vi "MenuSelection(User).vi"(6 "User events":T8, 7 "Clipboard":refnum<vi>, 8 "error in":errorcluster {"code" min=0 max=0}, 10 "ItemTag":string, 11 "Data in":T1={"Class"={"Ants"=refnum, "Layer"=refnum, "Templates"=refnum, "Icon"=refnum, "Glyph"=refnum, "Settings"=refnum, "Tools"=refnum}, "Ref"={"Add Layer"=refnum, "Remove Layer"=refnum, "Line Text"=[], "Body Text Spec"=refnum, "DNL_Font"=refnum, "glyph path str"=refnum, "templates path str"=refnum, "Arrow Up"=refnum, "Arrow Down"=refnum, "IE VI Ref"=refnum, "Glyphs tree"=refnum, "Templates tree"=refnum, "Layer Icon Text"=refnum, "Layer Template"=refnum, "Body Text"=refnum, "Search Templates"=refnum, "TextMarker"=refnum, "Tab Control"=refnum, "Search Glyphs"=refnum, "Line Color"=refnum, "DNL_Glyphs []"=refnum, "Fill Color"=refnum, "Tools"=refnum, "Icon"=refnum, "Preview"=refnum, "Ants"=refnum, "Terminals"=refnum, "menu reference"=refnum, "LayerNames"=[], "GlyphLoadAnimation"=refnum, "TemplateLoadAnimation"=refnum, "refreshGlyphs"=refnum, "refreshTemplates"=refnum}, "Support"={"AntsRect"={"left"=0, "top"=0, "right"=0, "bottom"=0}, "Mouse Move Coords"={"Horizontal"=0, "Vertical"=0}, "Mouse Down Coords"={"Horizontal"=0, "Vertical"=0}, "Temp Coord"={"Horizontal"=0, "Vertical"=0}, "Action"=enum."Default", "Edge Color"=4914962, "Fill Color"=16860, "Mouse Down?"=FALSE, "Draft Mode?"=FALSE, "Temp Icon"=bytes[3102], "CTRL Pressed"=FALSE, "Move Selection?"=FALSE, "AntsRect Orig"={"left"=0, "top"=0, "right"=0, "bottom"=0}, "Text"="", "TM Set?"=FALSE, "Mouse inside icon?"=FALSE, "Tool (old value)"=0, "Pencil Move Color"=0, "Swap Colors?"=FALSE, "Shift pressed?"=FALSE}}) -> (0 "error out":errorcluster {"code" min=0 max=0}, 3 "Data out":T1={"Class"={"Ants"=refnum, "Layer"=refnum, "Templates"=refnum, "Icon"=refnum, "Glyph"=refnum, "Settings"=refnum, "Tools"=refnum}, "Ref"={"Add Layer"=refnum, "Remove Layer"=refnum, "Line Text"=[], "Body Text Spec"=refnum, "DNL_Font"=refnum, "glyph path str"=refnum, "templates path str"=refnum, "Arrow Up"=refnum, "Arrow Down"=refnum, "IE VI Ref"=refnum, "Glyphs tree"=refnum, "Templates tree"=refnum, "Layer Icon Text"=refnum, "Layer Template"=refnum, "Body Text"=refnum, "Search Templates"=refnum, "TextMarker"=refnum, "Tab Control"=refnum, "Search Glyphs"=refnum, "Line Color"=refnum, "DNL_Glyphs []"=refnum, "Fill Color"=refnum, "Tools"=refnum, "Icon"=refnum, "Preview"=refnum, "Ants"=refnum, "Terminals"=refnum, "menu reference"=refnum, "LayerNames"=[], "GlyphLoadAnimation"=refnum, "TemplateLoadAnimation"=refnum, "refreshGlyphs"=refnum, "refreshTemplates"=refnum}, "Support"={"AntsRect"={"left"=0, "top"=0, "right"=0, "bottom"=0}, "Mouse Move Coords"={"Horizontal"=0, "Vertical"=0}, "Mouse Down Coords"={"Horizontal"=0, "Vertical"=0}, "Temp Coord"={"Horizontal"=0, "Vertical"=0}, "Action"=enum."Default", "Edge Color"=4914962, "Fill Color"=16860, "Mouse Down?"=FALSE, "Draft Mode?"=FALSE, "Temp Icon"=bytes[3102], "CTRL Pressed"=FALSE, "Move Selection?"=FALSE, "AntsRect Orig"={"left"=0, "top"=0, "right"=0, "bottom"=0}, "Text"="", "TM Set?"=FALSE, "Mouse inside icon?"=FALSE, "Tool (old value)"=0, "Pencil Move Color"=0, "Swap Colors?"=FALSE, "Shift pressed?"=FALSE}})   [LabVIEW 2021]
uses:
  <resource>/plugins/NIIconEditor/Controls/Global Data.ctl
  <resource>/plugins/NIIconEditor/Class/Ants/Ants.lvclass
  <resource>/plugins/NIIconEditor/Class/FakedArray/FakedArray.lvclass
  <vilib>/LabVIEW Icon API/lv_icon/Classes/Icon/Icon.lvclass
  <resource>/plugins/NIIconEditor/Class/Icon Library/Glyph.lvclass
  <resource>/plugins/NIIconEditor/Class/Settings/Settings.lvclass
  <resource>/plugins/NIIconEditor/Class/Tools/Tools Paint.lvclass
  <resource>/plugins/NIIconEditor/Controls/IE Classes.ctl
  <resource>/plugins/NIIconEditor/Controls/References Cluster.ctl
  <resource>/plugins/NIIconEditor/Controls/SupportClass.ctl
  <vilib>/Utility/miscctls.llb/LVPoint32TypeDef.ctl
  <resource>/plugins/NIIconEditor/Controls/SupportClass_Action.ctl
  <vilib>/LabVIEW Icon API/lv_icon/Controls/IEColor.ctl
  <vilib>/LabVIEW Icon API/lv_icon/Controls/Pathes.ctl
  <vilib>/LabVIEW Icon API/lv_icon/Controls/Graphic.ctl
  <vilib>/LabVIEW Icon API/lv_icon/Classes/Icon Framework/Icon Framework.lvclass
  <vilib>/LabVIEW Icon API/lv_icon/Classes/Layer/Layer.lvclass
  <vilib>/LabVIEW Icon API/lv_icon/Controls/Layer.ctl
  <resource>/plugins/NIIconEditor/Controls/Undo Redo Action.ctl
  <resource>/plugins/NIIconEditor/Controls/Tools.ctl
  <vilib>/LabVIEW Icon API/lv_icon/lv_icon.lvlib
panel:
  in  "Layer name":string="Clipboard"
  in  "glyph":string="Glyph name"
  in  "template":string="Template name"
  in  "Prompt":string="Save Glyph"
  in  "prompt":string="Save Icon Template"
  in  "LayerName":string="Merged Layers"
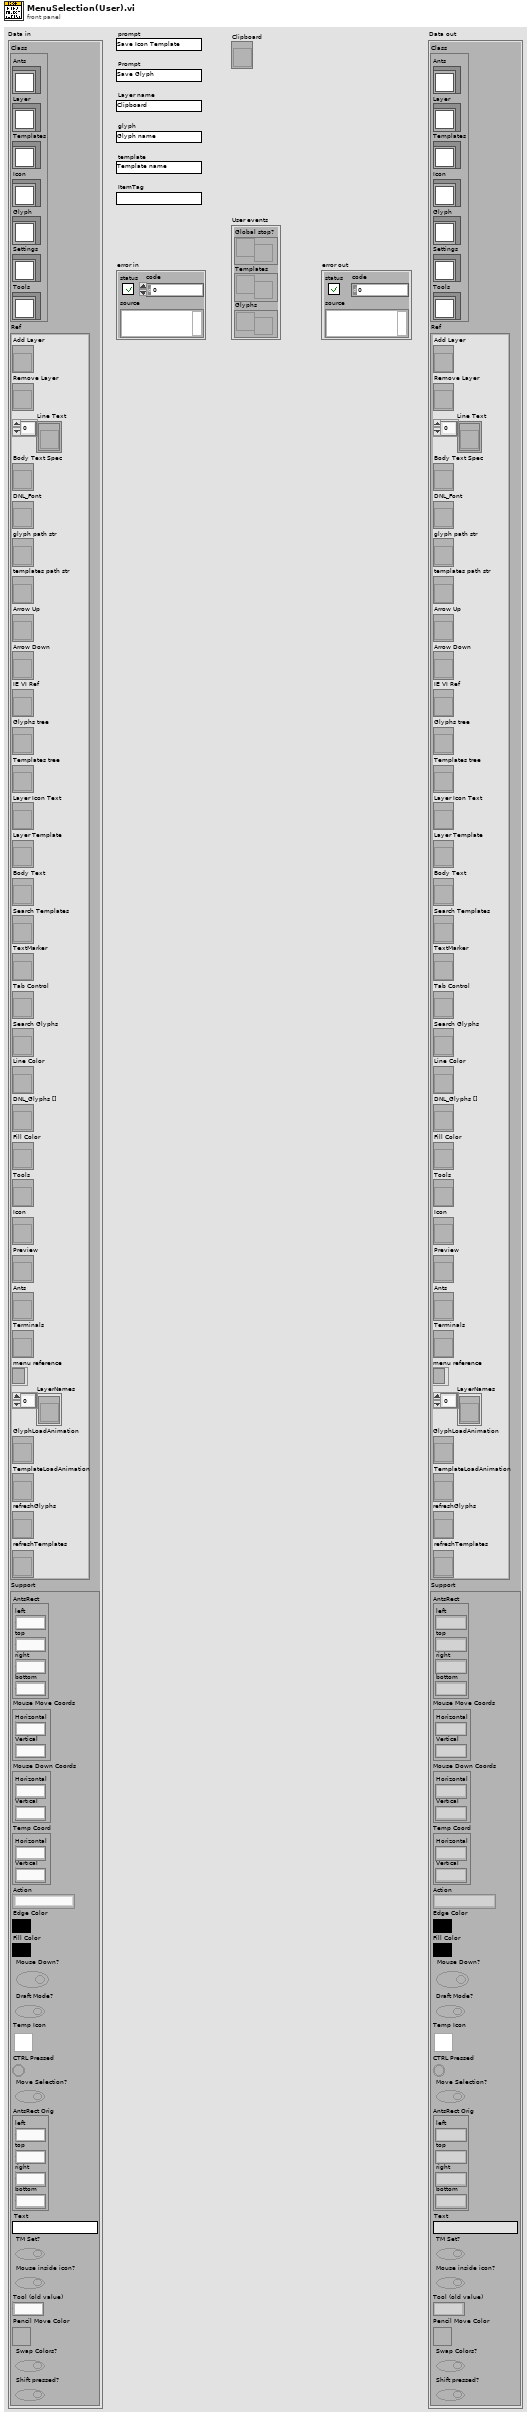
[diagram p1: front panel]
types:
  T1 = typedef "lv_icon.lvlib/Global Data.ctl" = cluster{"Class":T2, "Ref":T3, "Support":T4}
  T2 = typedef "IE Classes.ctl" = cluster{"Ants":refnum<class "Ants.lvclass">, "Layer":refnum<class "FakedArray.lvclass">, "Templates":refnum<class "FakedArray.lvclass">, "Icon":refnum<class "Icon.lvclass">, "Glyph":refnum<class "Glyph.lvclass">, "Settings":refnum<class "Settings.lvclass">, "Tools":refnum<class "Tools Paint.lvclass">}
  T3 = typedef "lv_icon.lvlib/References Cluster.ctl" = cluster{"Add Layer":refnum<vi>, "Remove Layer":refnum<vi>, "Line Text":refnum<vi>[], "Body Text Spec":refnum<vi>, "DNL_Font":refnum<vi>, "glyph path str":refnum<vi>, "templates path str":refnum<vi>, "Arrow Up":refnum<vi>, "Arrow Down":refnum<vi>, "IE VI Ref":refnum<vi>, "Glyphs tree":refnum<vi>, "Templates tree":refnum<vi>, "Layer Icon Text":refnum<vi>, "Layer Template":refnum<vi>, "Body Text":refnum<vi>, "Search Templates":refnum<vi>, "TextMarker":refnum<vi>, "Tab Control":refnum<vi>, "Search Glyphs":refnum<vi>, "Line Color":refnum<vi>, "DNL_Glyphs []":refnum<vi>, "Fill Color":refnum<vi>, "Tools":refnum<vi>, "Icon":refnum<vi>, "Preview":refnum<vi>, "Ants":refnum<vi>, "Terminals":refnum<vi>, "menu reference":refnum<k9>, "LayerNames":refnum<vi>[], "GlyphLoadAnimation":refnum<vi>, "TemplateLoadAnimation":refnum<vi>, "refreshGlyphs":refnum<vi>, "refreshTemplates":refnum<vi>}
  T4 = typedef "SupportClass.ctl" = cluster{"AntsRect":cluster{"left":i16, "top":i16, "right":i16, "bottom":i16}, "Mouse Move Coords":T5, "Mouse Down Coords":T5, "Temp Coord":T5, "Action":T6, "Edge Color":T7, "Fill Color":T7, "Mouse Down?":bool, "Draft Mode?":bool, "Temp Icon":picture, "CTRL Pressed":bool, "Move Selection?":bool, "AntsRect Orig":cluster{"left":i16, "top":i16, "right":i16, "bottom":i16}, "Text":string, "TM Set?":bool, "Mouse inside icon?":bool, "Tool (old value)":u32, "Pencil Move Color":u32, "Swap Colors?":bool, "Shift pressed?":bool}
  T5 = typedef "LVPoint32TypeDef.ctl" = cluster{"Horizontal":i32, "Vertical":i32}
  T6 = typedef "SupportClass_Action.ctl" = enum16{"Default", "Move Selection", "Glyph Library", "Tool"}
  T7 = typedef "IEColor.ctl" = u32
  T8 = cluster{"Global stop?":refnum<user-event>, "Templates":refnum<user-event>, "Glyphs":refnum<user-event>}
  T9 = typedef "Pathes.ctl" = enum16{"Root Path", "Icon Templates", "Icon Templates VI", "Icon Templates Lib", "Glyphs"}
  T10 = typedef "Graphic.ctl" = cluster{"Rectangle":cluster{"left":i16, "top":i16, "right":i16, "bottom":i16}, "Path":path, "Image":picture, "Filter":string, "FileName":string}
  T11 = typedef "Layer.ctl" = cluster{"LayerIcon":picture, "LayerName":string, "Opacity":u8, "Visibility?":bool}
  T12 = typedef "Undo Redo Action.ctl" = enum16{"Init", "Add", "Undo", "Redo", "Current State"}
  T13 = enum32{"Pencil", "Line", "Dropper", "Fill", "Rectangle", "Filled Rectangle", "Ellipse", "Filled Ellipse", "Eraser", "Text", "Select", "Move"}
  T14 = typedef "Tools.ctl" = enum32{"Pencil", "Line", "Dropper", "Fill", "Rectangle", "Filled Rectangle", "Ellipse", "Filled Ellipse", "Eraser", "Text", "Select", "Move"}
  T15 = typedef "imagedata.ctl" = cluster{"image type":i32, "image depth":i32, "image":u8[], "mask":u8[], "colors":u32[], "Rectangle":cluster{"left":i16, "top":i16, "right":i16, "bottom":i16}}
  T16 = typedef "Font.ctl" = string
  T17 = typedef "Alignment.ctl" = u16
  T18 = typedef "Font Size.ctl" = u8
  T19 = cluster{"Line 1 text":string, "Line 2 text":string, "Line 3 text":string, "Line 4 text":string, "Line 1 color":u32, "Line 2 color":u32, "Line 3 color":u32, "Line 4 color":u32, "Body Text Spec":cluster{"DNL_Font":T16, "Alignment":T17, "Size":T18}, "Center text vertically":bool, "Capitalize Text":bool}
  T20 = cluster{"left":i16, "top":i16, "right":i16, "bottom":i16}
  T21 = cluster{"Horizontal":i32, "Vertical":i32, "Vertical 2":i32, "Vertical 3":i32}
  T22 = cluster{"Left":i32, "Top":i32, "Right":i32, "Bottom":i32}
  T23 = typedef "Icon Editor Invoker Type.ctl" = enum32{"Unknown Icon Source", "VI Icon", "Library Icon (any library type)", "Palette icon", "Icon from App Method"}
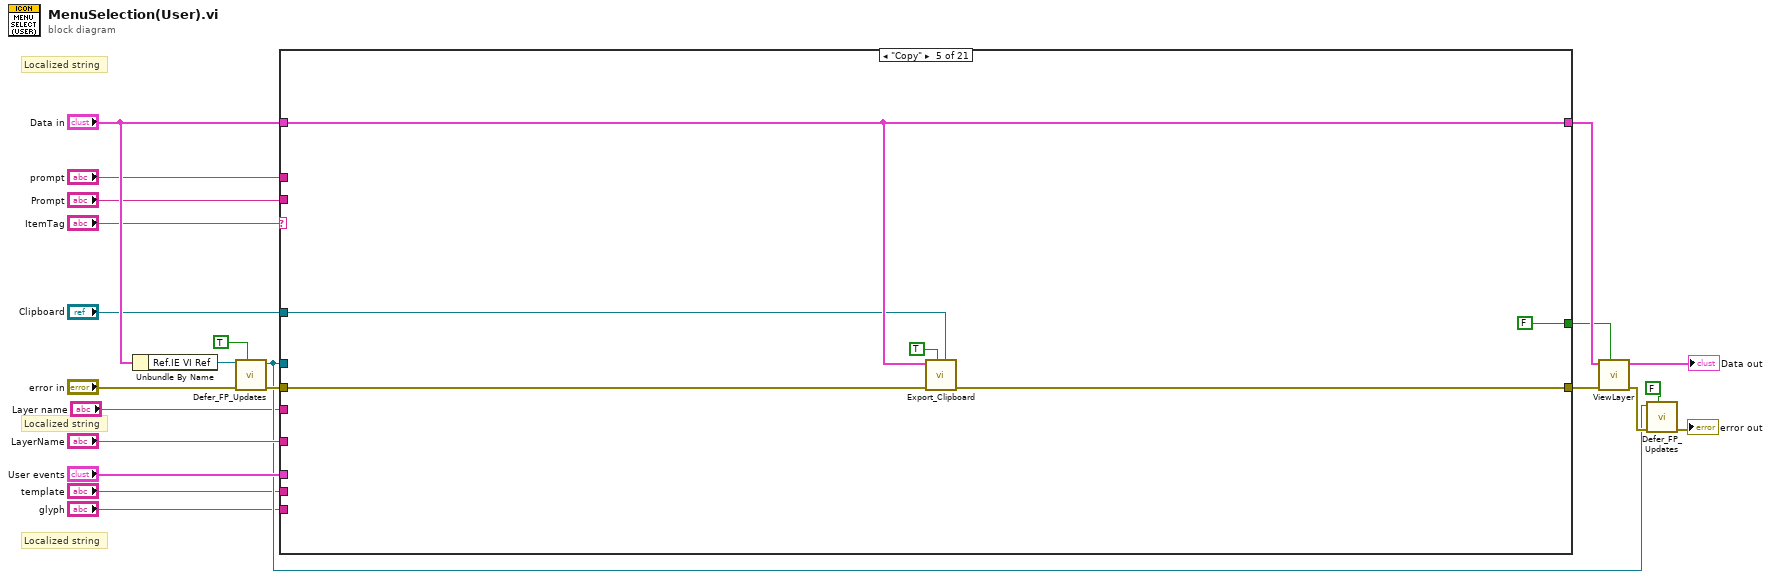
[diagram p0: block diagram]
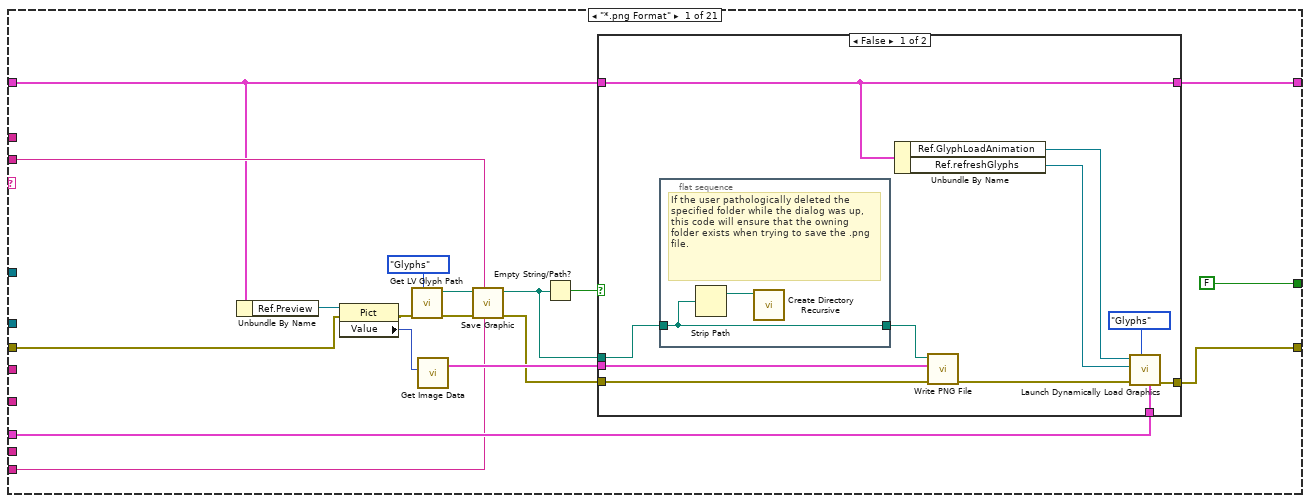
[diagram p2: hidden frame]
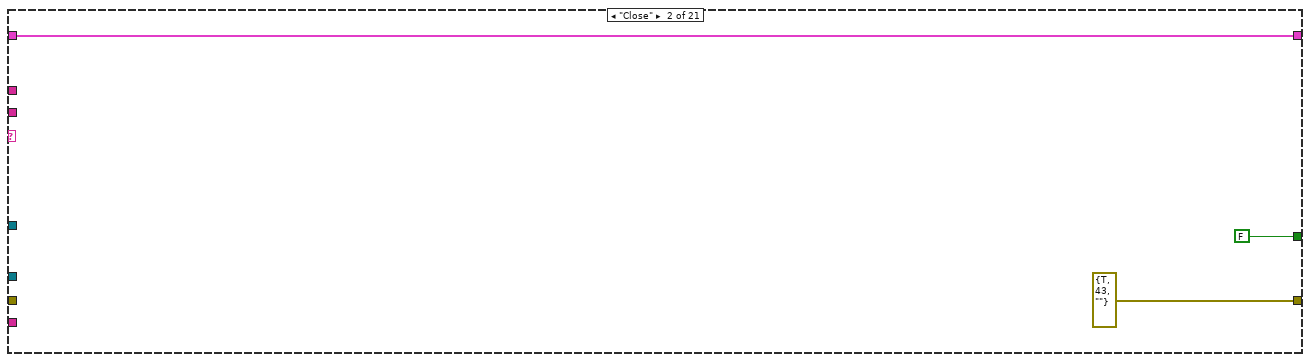
[diagram p4: hidden frame]
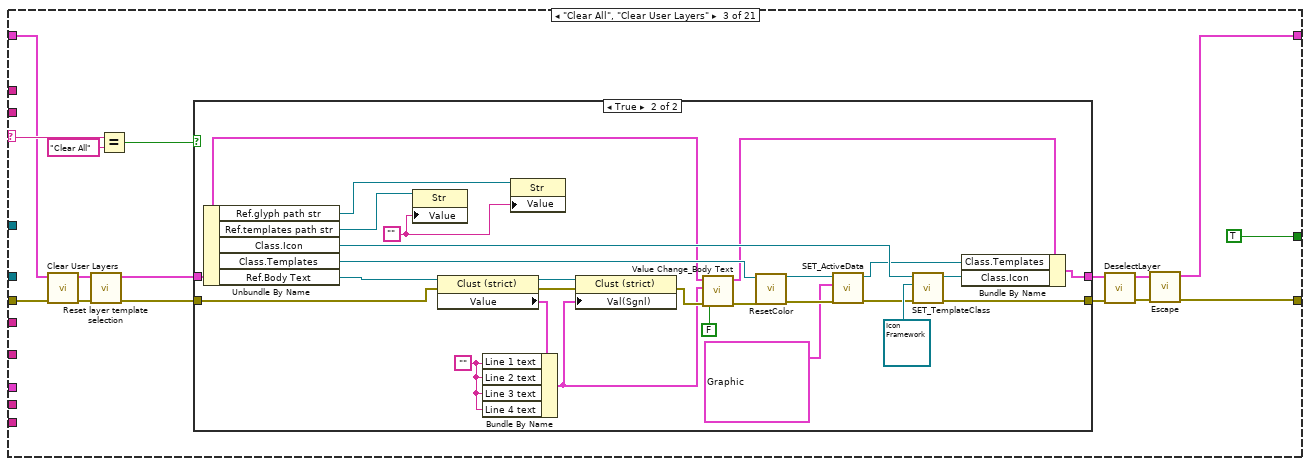
[diagram p5: hidden frame]
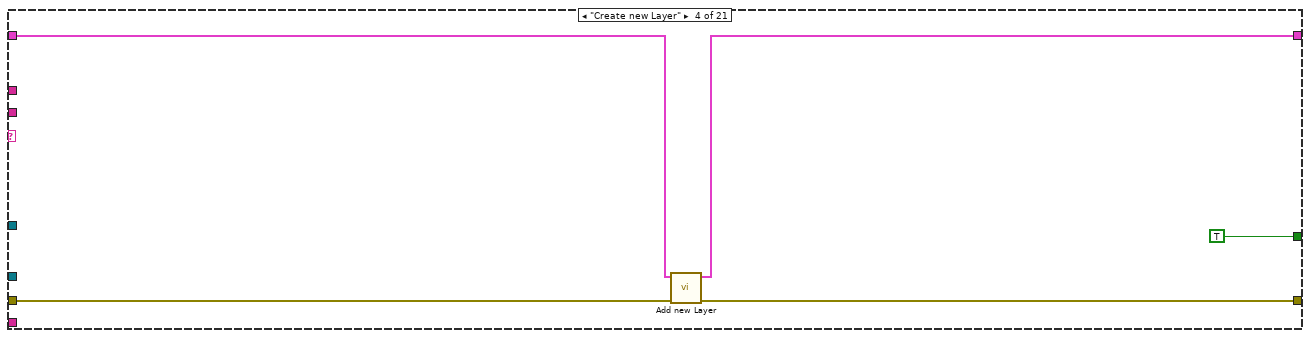
[diagram p7: hidden frame]
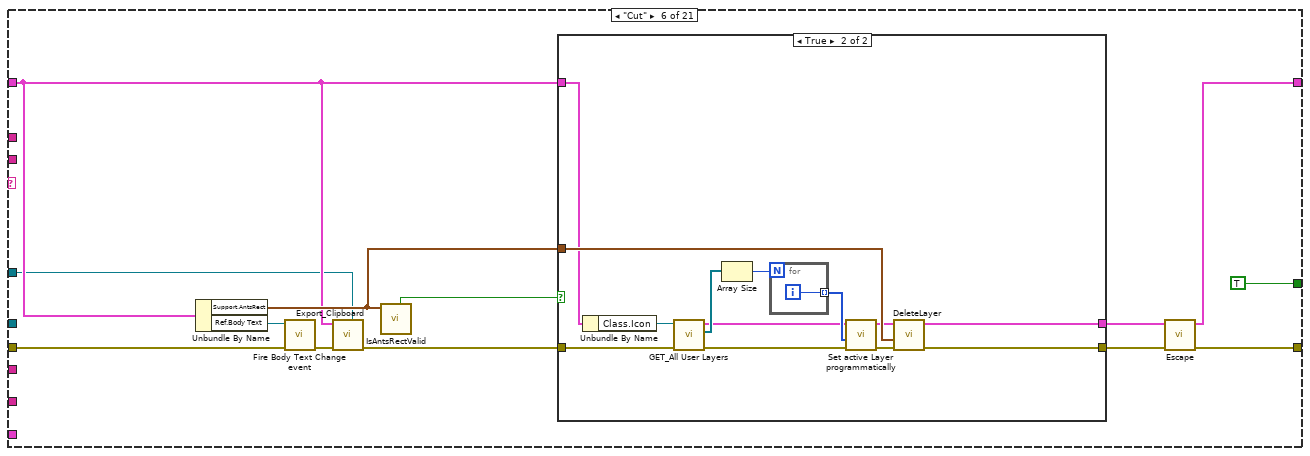
[diagram p8: hidden frame]
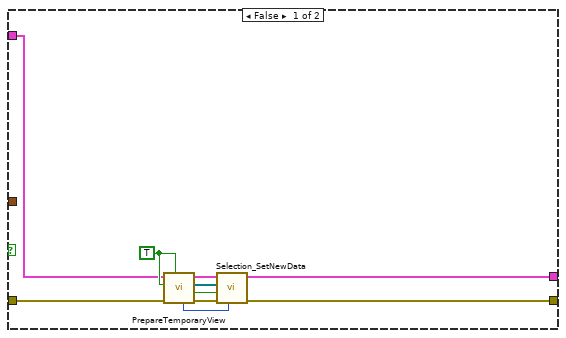
[diagram p9: hidden frame]
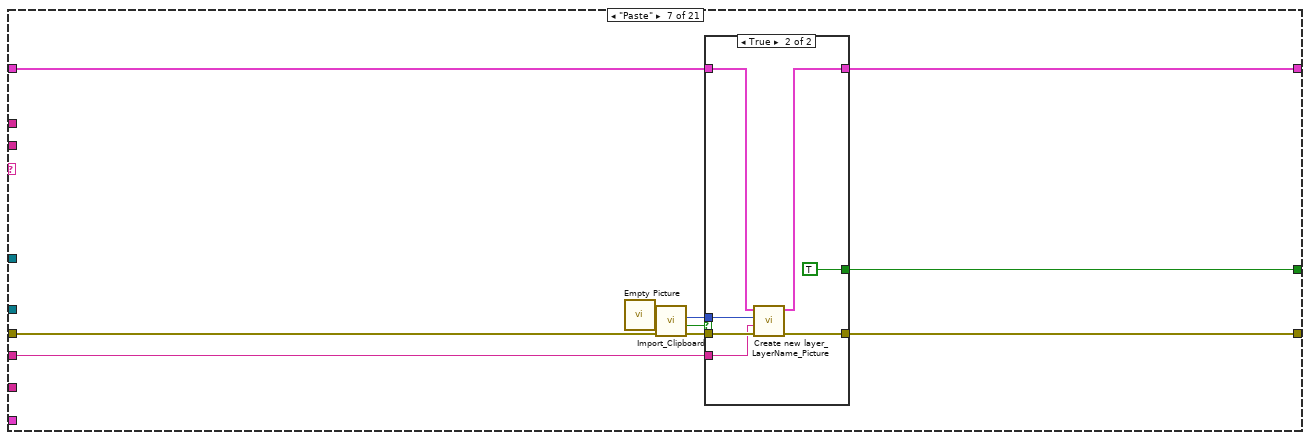
[diagram p10: hidden frame]
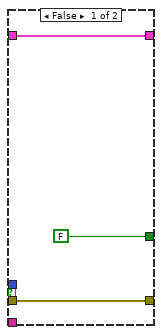
[diagram p11: hidden frame]
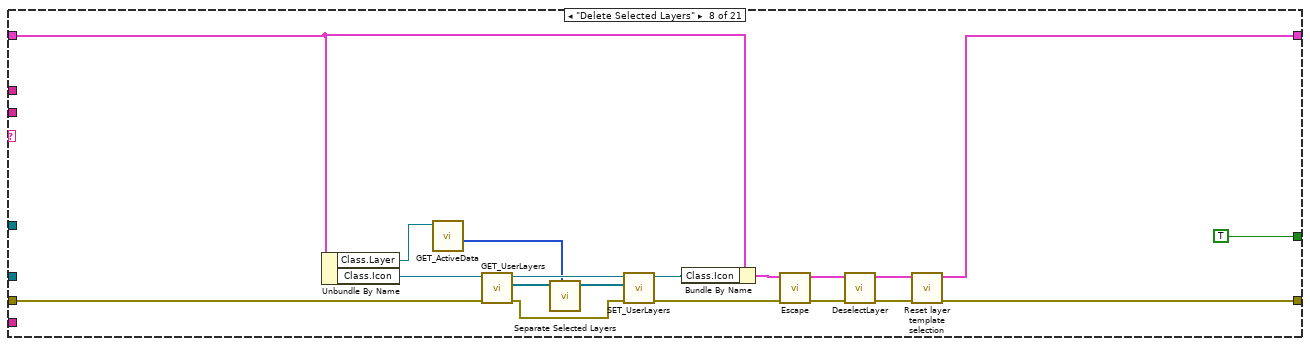
[diagram p12: hidden frame]
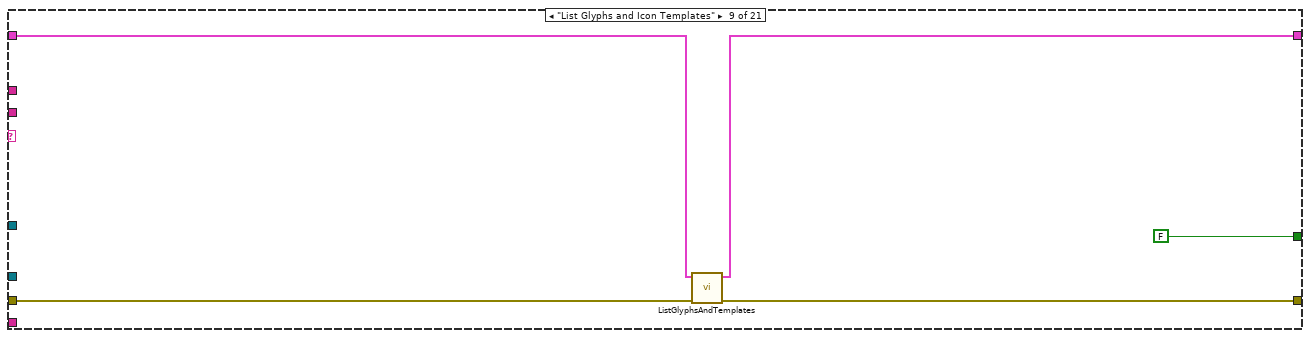
[diagram p13: hidden frame]
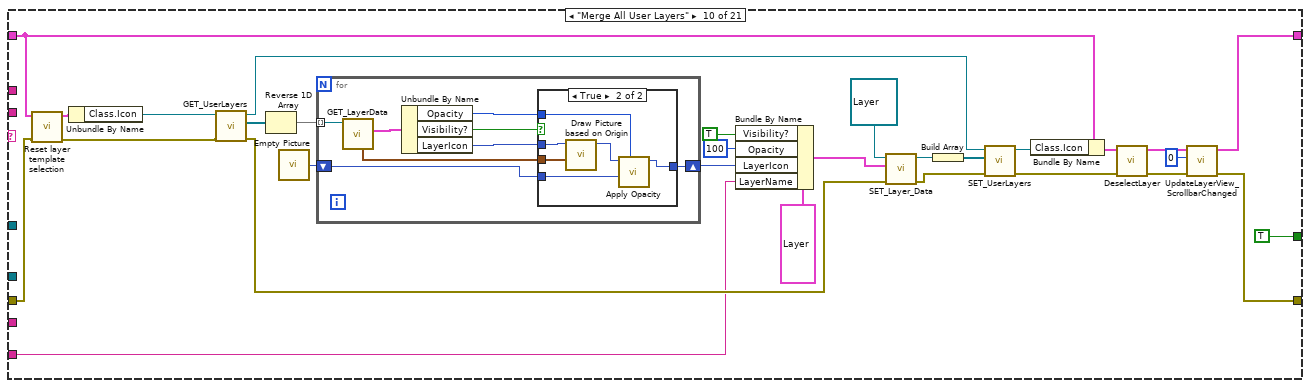
[diagram p14: hidden frame]
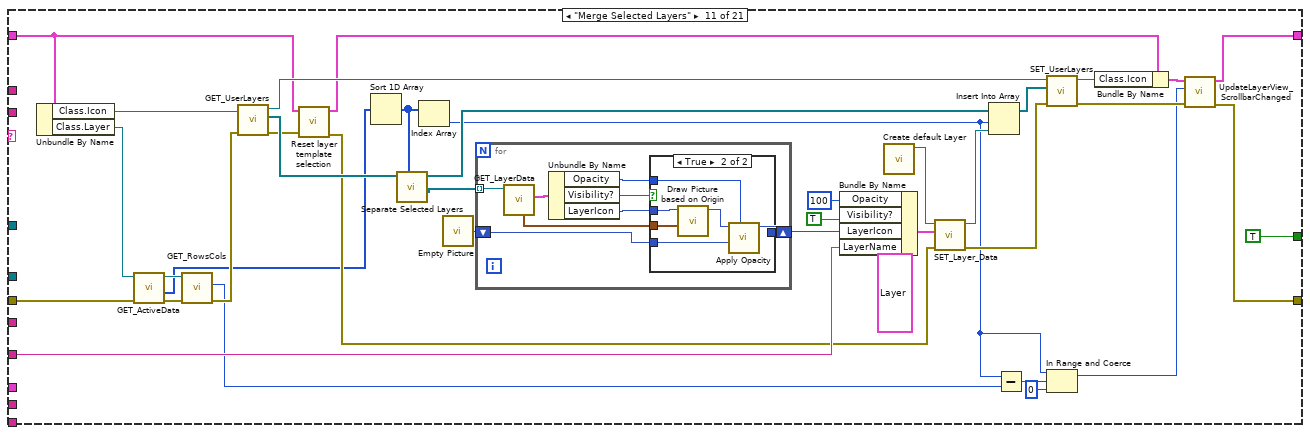
[diagram p16: hidden frame]
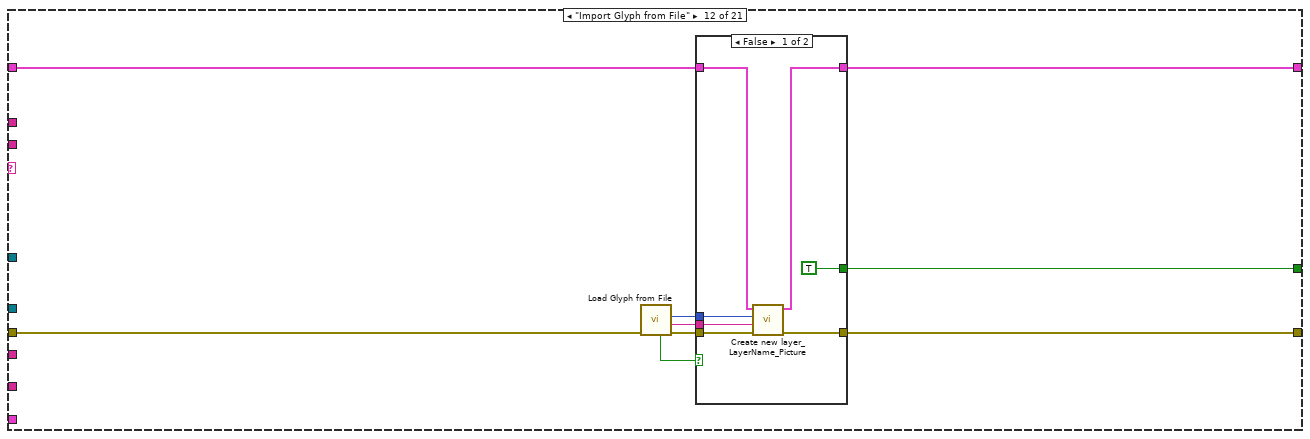
[diagram p18: hidden frame]
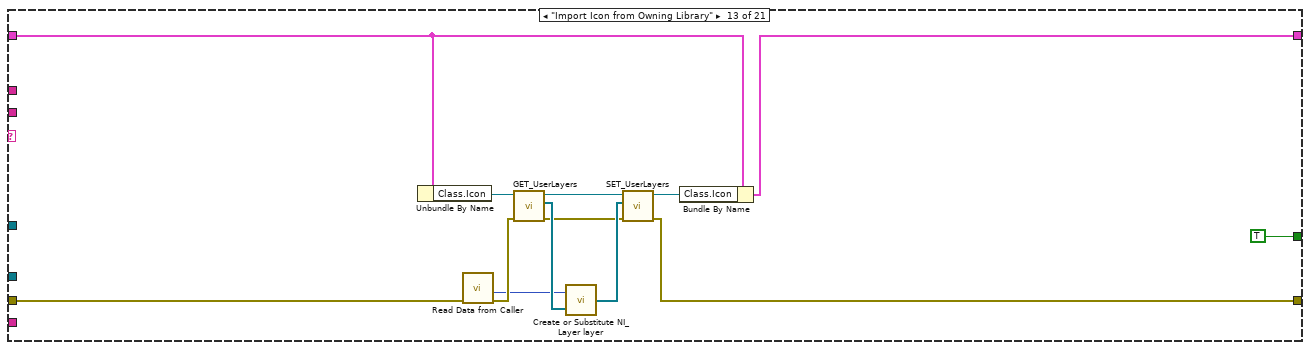
[diagram p20: hidden frame]
diagram:
  # "Localized string"
  # "Localized string"
  # "Localized string"
  n1 = Unbundle By Name("Data in") -> ("Ref.IE VI Ref"=w9:refnum<vi>)
  n2 = call <resource>:"Defer_FP_Updates.vi"("Defer Panel Updates"=TRUE, "error in (no error)"="error in", "lv_icon.vi in"=w9) -> ("error out"=w11:errorcluster, "lv icon.vi out"=w5:refnum<vi>)  [unwired: 7 out]
  n3 = case shown="\"Copy\"" "ItemTag" {
    selector: "ItemTag" -> [_ _ w74 _ _ _ _ _ _ _ _ _ _ w340 _ w388 _ _ _ _ _]
    tunnel: w11 -> [w27 _ w63 w103 w113 w118 w154 w180 w193 w208 w239 w296 w321 w325 w373 w378 w397 w399 w422 w445 w477]
    tunnel: [w28 errorcluster {"status"=TRUE, "code"=43, "source"=""} ("Icon 43") w66 w104 w112 w125 w157 w170 w192 w195 w251 w298 w312 w331 w354 w380 w390 w400 w429 w444 w477] -> w16
    tunnel: "LayerName" -> [_ _ _ _ _ _ _ _ _ w210 w264 _ _ _ _ _ _ _ _ _ _]
    tunnel: "prompt" -> [_ _ _ _ _ _ _ _ _ _ _ _ _ _ _ _ _ _ _ w447 _]
    tunnel: "Prompt" -> [w29 _ _ _ _ _ _ _ _ _ _ _ _ _ _ _ _ _ _ _ _]
    tunnel: [FALSE FALSE TRUE TRUE FALSE TRUE w159 TRUE FALSE TRUE TRUE w291 TRUE FALSE FALSE FALSE FALSE FALSE FALSE FALSE FALSE] -> w13
    tunnel: "User events" -> [w34 _ _ _ _ _ _ _ _ _ _ _ _ _ _ _ _ _ w427 w453 _]
    tunnel: [w23 w56 w67 w106 w109 w124 w156 w173 w189 w196 w253 w297 w309 w324 w355 w379 w389 w398 w413 w440 w475] -> w14
    tunnel: "Data in" -> [w24 w56 w64 w105 w109 w115 w158 w175 w190 w204 w256 w299 w311 w327 w369 w381 w396 w403 w414 w450 w475]
    tunnel: w5 -> [_ _ _ _ _ _ _ _ _ _ _ _ _ _ _ _ _ _ _ _ _]
    tunnel: "template" -> [_ _ _ _ _ _ _ _ _ _ _ _ _ _ _ _ _ _ _ w442 _]
    tunnel: "glyph" -> [w25 _ _ _ _ _ _ _ _ _ _ _ _ _ _ _ _ _ _ _ _]
    tunnel: "Layer name" -> [_ _ _ _ _ _ w150 _ _ _ _ _ _ _ _ _ _ _ _ _ _]
    tunnel: "Clipboard" -> [_ _ _ _ w108 w114 _ _ _ _ _ _ _ _ _ _ _ _ _ _ _]
    frame "*.png Format" {
      n4 = Unbundle By Name(w24) -> ("Ref.Preview"=w40:refnum<vi>)
      n5 = property class="Pict"(reference=w40, error in=w27) -> (error out=w36:errorcluster, "Value"=w38:picture)  [unwired: 1 out]
      n6 = call <vilib>:"Get LV Glyph Path.vi"("Path"=Pathes."Glyphs", "error in (no error)"=w36) -> ("error out"=w33:errorcluster, "Requested Path"=w30:path)  [unwired: 1 in, 7 out]
      n7 = call <vilib>:"Get Image Data.vi"("Pic In"=w38) -> ("image data out"=w39:T15)  [unwired: 3 in, 7 out]
      n8 = call <resource>:"Save Graphic.vi"("Loc string caption"=w25, "FP Title"=w29, "error in (no error)"=w33, "Start path in"=w30) -> ("error out"=w32:errorcluster, "Output"=w31:path)  [unwired: 6 out]
      n9 = Empty String/Path?(string/path=w31) -> (empty?=w26:bool)
      n10 = case shown="False" w26 {
        tunnel: w39 -> [w51 _]
        tunnel: w34 -> [w48 _]
        tunnel: w32 -> [w47 w55]
        tunnel: w31 -> [w42 _]
        tunnel: [w46 w55] -> w28
        tunnel: w24 -> [w45 w54]
        tunnel: [w45 w54] -> w23
        frame False {
          n11 = flat-sequence {
            tunnel: w42 -> [w53]
            tunnel: [w53] -> w41
            frame #0 {
              # "If the user pathologically deleted the specified folder while the dialog was up, this code will ensure that the owning folder exists when trying to save the .png file."
              n12 = Strip Path(path=w53) -> (stripped path=w52:path)  [unwired: 1 out]
              n13 = call <vilib>:"Create Directory Recursive.vi"("directory"=w52) -> ()  [unwired: 4 in, 3 out]
            }
          }
          n14 = Unbundle By Name(w45) -> ("Ref.GlyphLoadAnimation"=w43:refnum<vi>, "Ref.refreshGlyphs"=w44:refnum<vi>)
          n15 = call <vilib>:"Write PNG File.vi"("error in (no error)"=w47, "image data"=w51, "path to PNG file"=w41) -> ("error out"=w50:errorcluster)  [unwired: 1 in, 7 out]
          n16 = call <resource>:"Launch Dynamically Load Graphics.vi"("User events"=w48, "Path"=Pathes."Glyphs", "error in (no error)"=w50, "button ref"=w44, "animatedDecoration ref"=w43) -> ("error out"=w46:errorcluster)  [unwired: 1 in, 5 out]
        }
        frame True {
        }
      }
    }
    frame "Close" {
    }
    frame "Clear All", "Clear User Layers" {
      n17 = call <resource>:"Clear User Layers.vi"("error in"=w63, "Data in"=w64) -> ("error out"=w62:errorcluster, "Data out"=w61:T1)  [unwired: 8 out]
      n18 = call <resource>:"Reset layer template selection.vi"("error in (no error)"=w62, "Data in"=w61) -> ("error out"=w59:errorcluster, "Data out"=w60:T1)  [unwired: 1 in, 7 out]
      n19 = Equal?(x=w74, y="Clear All") -> (x = y?=w73:bool)
      n20 = case shown="True" w73 {
        tunnel: w59 -> [w76 w90]
        tunnel: w60 -> [w75 w81]
        tunnel: [w76 w84] -> w71
        tunnel: [w75 w82] -> w69
        frame False {
        }
        frame True {
          w77 = ""
          w98 = ""
          n21 = Unbundle By Name(w81) -> ("Ref.glyph path str"=w78:refnum<vi>, "Ref.templates path str"=w79:refnum<vi>, "Class.Icon"=w87:refnum<class "Icon.lvclass">, "Class.Templates"=w89:refnum<class "FakedArray.lvclass">, "Ref.Body Text"=w102:refnum<vi>)
          n22 = property class="Str"(reference=w79, "Value"=w77) -> ()  [unwired: 1 in, 2 out]
          n23 = property class="Clust (strict)"(reference=w102, error in=w90) -> (reference out=w101:refnum<vi>, error out=w100:errorcluster, "Value"=w99:T19)
          n24 = Bundle By Name(cluster=w99, "Line 1 text"=w98, "Line 2 text"=w98, "Line 3 text"=w98, "Line 4 text"=w98) -> (w91:T19)
          n25 = property class="Str"(reference=w78, "Value"=w77) -> ()  [unwired: 1 in, 2 out]
          n26 = property class="Clust (strict)"(reference=w101, error in=w100, "Val(Sgnl)"=w91) -> (error out=w93:errorcluster)  [unwired: 1 out]
          n27 = call <resource>:"Value Change_Body Text.vi"("Add to Undo?"=FALSE, "error in"=w93, "NewVal"=w91, "Data in"=w81) -> ("error out"=w88:errorcluster, "Data out"=w80:T1)  [unwired: 1 in, 5 out]
          n28 = call <resource>:"ResetColor.vi"("error in (no error)"=w88, "FakedArray in"=w89) -> ("error out"=w96:errorcluster, "FakedArray out"=w97:refnum<class "FakedArray.lvclass">)  [unwired: 8 out]
          n29 = call-dynamic "SET_ActiveData.vi"("error in (no error)"=w96, "Active Data"=T10 {"Rectangle"={"left"=0, "top"=0, "right"=0, "bottom"=0}, "Path"=path "", "Image"=bytes[0], "Filter"="", "FileName"=""} ("Path & Icon"), "FakedArray.lvclass in"=w97) -> ("error out"=w86:errorcluster, "FakedArray.lvclass out"=w83:refnum<class "FakedArray.lvclass">)  [unwired: 7 out]
          n30 = call-dynamic "SET_TemplateClass.vi"("error in (no error)"=w86, "Icon Framework.lvclass"=refnum<class "Icon Framework.lvclass"> refnum ("lv_icon.lvlib:Icon Framework.lvclass"), "Icon.lvclass in"=w87) -> ("error out"=w84:errorcluster, "Icon.lvclass out"=w85:refnum<class "Icon.lvclass">)  [unwired: 7 out]
          n31 = Bundle By Name(cluster=w80, "Class.Templates"=w83, "Class.Icon"=w85) -> (w82:T1)
        }
      }
      n32 = call <resource>:"DeselectLayer.vi"("error in (no error)"=w71, "Data in"=w69) -> ("error out"=w65:errorcluster, "Data out"=w68:T1)  [unwired: 8 out]
      n33 = call <resource>:"Escape.vi"("error in"=w65, "Data in"=w68) -> ("error out"=w66:errorcluster, "Data out"=w67:T1)  [unwired: 2 in, 6 out]
    }
    frame "Create new Layer" {
      n34 = call <resource>:"Add new Layer.vi"("error in"=w103, "Data in"=w105) -> ("error out"=w104:errorcluster, "Data out"=w106:T1)  [unwired: 8 out]
    }
    frame "Copy" {
      n35 = call <resource>:"Export_Clipboard.vi"("Clipboard"=w108, "Is Copy? (F)"=TRUE, "error in"=w113, "Data in"=w109) -> ("error out"=w112:errorcluster)  [unwired: 1 in, 6 out]
    }
    frame "Cut" {
      n36 = Unbundle By Name(w115) -> ("Support.AntsRect"=w121:T20, "Ref.Body Text"=w119:refnum<vi>)
      n37 = call <resource>:"Fire Body Text Change event.vi"("error in"=w118, "Ref.Body Text"=w119) -> ("error out"=w117:errorcluster)  [unwired: 2 in, 7 out]
      n38 = call <resource>:"Export_Clipboard.vi"("Clipboard"=w114, "error in"=w117, "Data in"=w115) -> ("error out"=w122:errorcluster)  [unwired: 1 in, 7 out]
      n39 = call <resource>:"IsAntsRectValid.vi"("AntsRect"=w121) -> ("Max. Rect size?"=w123:bool)  [unwired: 10 out]
      n40 = case shown="True" w123 {
        tunnel: [w136 w147] -> w116
        tunnel: [w135 w148] -> w120
        tunnel: w122 -> [w128 w139]
        tunnel: w121 -> [_ w146]
        tunnel: w115 -> [w127 w137]
        frame False {
          w134 = TRUE ("Delete Selected Area?")
          n41 = call <resource>:"PrepareTemporaryView.vi"("Delete Selected Area?"=w134, "error in (no error)"=w128, "Valid Selection?"=w134, "Data in"=w127) -> ("error out"=w131:errorcluster, "Highlighted?"=w132:bool, "All Layers out"=w133:refnum<class "Layer.lvclass">[], "Data out"=w129:T1, "#Active Layer"=w130:i32)  [unwired: 1 in, 2 out]
          n42 = call <resource>:"Selection_SetNewData.vi"("#Active Layer"=w130, "error in"=w131, "Highlighted?"=w132, "All Layers In"=w133, "Data in"=w129) -> ("error out"=w136:errorcluster, "Data out"=w135:T1)  [unwired: 1 in, 3 out]
        }
        frame True {
          n43 = Unbundle By Name(w137) -> ("Class.Icon"=w145:refnum<class "Icon.lvclass">)
          n44 = call-dynamic "GET_All User Layers.vi"("error in (no error)"=w139, "Icon.lvclass in"=w145) -> ("error out"=w144:errorcluster, "User Layer"=w141:refnum<class "Layer.lvclass">[])  [unwired: 7 in, 1 out]
          n45 = Array Size(array=w141) -> (size(s)=w142:i32)
          n46 = for {
            N: w142 -> [_]
            tunnel: [w149] -> w143 mode=indexing
            i -> [w149]
          }
          n47 = call <resource>:"Set active Layer programmatically.vi"("error in"=w144, "Active Layer []"=w143, "Data in"=w137) -> ("error out"=w138:errorcluster, "Data out"=w140:T1)  [unwired: 7 in]
          n48 = call <resource>:"DeleteLayer.vi"("error in"=w138, "AntsRect"=w146, "Data in"=w140) -> ("error out"=w147:errorcluster, "Data out"=w148:T1)  [unwired: 5 out]
        }
      }
      n49 = call <resource>:"Escape.vi"("error in"=w116, "Data in"=w120) -> ("error out"=w125:errorcluster, "Data out"=w124:T1)  [unwired: 2 in, 6 out]
    }
    frame "Paste" {
      n50 = call "Empty Picture"() -> ("empty picture"=w155:picture)
      n51 = call <resource>:"Import_Clipboard.vi"("error in (no error)"=w154, "Picture in"=w155) -> ("error out"=w153:errorcluster, "Valid?"=w152:bool, "Picture"=w151:picture)  [unwired: 1 in, 6 out]
      n52 = case shown="True" w152 {
        tunnel: [FALSE TRUE] -> w159
        tunnel: w158 -> [w161 w169]
        tunnel: [w162 w168] -> w157
        tunnel: [w161 w167] -> w156
        tunnel: w153 -> [w162 w166]
        tunnel: w151 -> [_ w165]
        tunnel: w150 -> [_ w163]
        frame False {
        }
        frame True {
          n53 = call <resource>:"Create new layer_LayerName_Picture.vi"("error in"=w166, "Layer name"=w163, "Picture"=w165, "Data in"=w169) -> ("error out"=w168:errorcluster, "Data out"=w167:T1)  [unwired: 6 in]
        }
      }
    }
    frame "Delete Selected Layers" {
      n54 = Unbundle By Name(w175) -> ("Class.Layer"=w172:refnum<class "FakedArray.lvclass">, "Class.Icon"=w183:refnum<class "Icon.lvclass">)
      n55 = call-dynamic "GET_ActiveData.vi"("FakedArray in"=w172) -> ("Active Data []"=w181:i32[])  [unwired: 1 in, 9 out]
      n56 = call-dynamic "GET_UserLayers.vi"("error in (no error)"=w180, "Icon.lvclass in"=w183) -> ("error out"=w184:errorcluster, "All Layers"=w188:refnum<class "Layer.lvclass">[], "Icon.lvclass out"=w187:refnum<class "Icon.lvclass">)  [unwired: 7 out]
      n57 = call <resource>:"Separate Selected Layers.vi"("Active Indices"=w181, "All Layers"=w188) -> ("Layers out not in Array"=w186:refnum<class "Layer.lvclass">[])  [unwired: 9 out]
      n58 = call-dynamic "SET_UserLayers.vi"("error in (no error)"=w184, "Layers"=w186, "Icon.lvclass in"=w187) -> ("error out"=w171:errorcluster, "Icon.lvclass out"=w182:refnum<class "Icon.lvclass">)  [unwired: 7 in]
      n59 = Bundle By Name(cluster=w175, "Class.Icon"=w182) -> (w174:T1)
      n60 = call <resource>:"Escape.vi"("error in"=w171, "Data in"=w174) -> ("error out"=w179:errorcluster, "Data out"=w178:T1)  [unwired: 8 out]
      n61 = call <resource>:"DeselectLayer.vi"("error in (no error)"=w179, "Data in"=w178) -> ("error out"=w176:errorcluster, "Data out"=w177:T1)  [unwired: 8 out]
      n62 = call <resource>:"Reset layer template selection.vi"("error in (no error)"=w176, "Data in"=w177) -> ("error out"=w170:errorcluster, "Data out"=w173:T1)  [unwired: 1 in, 7 out]
    }
    frame "List Glyphs and Icon Templates" {
      n63 = call <resource>:"ListGlyphsAndTemplates.vi"("error in"=w193, "Data in"=w190) -> ("error out"=w192:errorcluster, "Data out"=w189:T1)  [unwired: 8 out]
    }
    frame "Merge All User Layers" {
      n64 = call <resource>:"Reset layer template selection.vi"("error in (no error)"=w208, "Data in"=w204) -> ("error out"=w207:errorcluster, "Data out"=w206:T1)  [unwired: 1 in, 7 out]
      n65 = Unbundle By Name(w206) -> ("Class.Icon"=w205:refnum<class "Icon.lvclass">)
      n66 = call-dynamic "GET_UserLayers.vi"("error in (no error)"=w207, "Icon.lvclass in"=w205) -> ("error out"=w214:errorcluster, "All Layers"=w222:refnum<class "Layer.lvclass">[], "Icon.lvclass out"=w221:refnum<class "Icon.lvclass">)  [unwired: 7 out]
      n67 = Reverse 1D Array(array=w222) -> (reversed array=w212:refnum<class "Layer.lvclass">[])
      n68 = call "Empty Picture"() -> ("empty picture"=w211:picture)
      n69 = for {
        shift-right: [w227] -> w218
        shift-left: w211 -> [w228]
        tunnel: w212 -> [w223] mode=indexing
        n70 = call-dynamic "GET_LayerData.vi"("Layer.lvclass in"=w223) -> ("Data"=w225:T11, "Origin"=w224:T5)  [unwired: 1 in, 8 out]
        n71 = Unbundle By Name(w225) -> ("Opacity"=w229:u8, "Visibility?"=w230:bool, "LayerIcon"=w226:picture)
        n72 = case shown="True" w230 {
          tunnel: w229 -> [_ w237]
          tunnel: w228 -> [w231 w236]
          tunnel: [w231 w235] -> w227
          tunnel: w226 -> [_ w234]
          tunnel: w224 -> [_ w233]
          frame False {
          }
          frame True {
            n73 = call <vilib>:"Draw Picture based on Origin.vi"("Origin"=w233, "LayerIcon in"=w234) -> ("LayerIcon out"=w232:picture)  [unwired: 1 in, 8 out]
            n74 = call <vilib>:"Apply Opacity.vi"("% (100)"=w237, "Bottom"=w236, "Top"=w232) -> ("new picture"=w235:picture)  [unwired: 8 out]
          }
        }
      }
      n75 = Bundle By Name(cluster=T11 {"LayerIcon"=bytes[0], "LayerName"="", "Opacity"=0, "Visibility?"=FALSE} ("Data"), "Visibility?"=TRUE, "Opacity"=u8 100, "LayerIcon"=w218, "LayerName"=w210) -> (w217:T11)
      n76 = call-dynamic "SET_Layer_Data.vi"("error in (no error)"=w214, "Data"=w217, "Layer.lvclass in"=refnum<class "Layer.lvclass"> refnum) -> ("error out"=w215:errorcluster, "Layer.lvclass out"=w220:refnum<class "Layer.lvclass">)  [unwired: 1 in, 6 out]
      n77 = Build Array(w220) -> (w213:refnum<class "Layer.lvclass">[])
      n78 = call-dynamic "SET_UserLayers.vi"("error in (no error)"=w215, "Layers"=w213, "Icon.lvclass in"=w221) -> ("error out"=w202:errorcluster, "Icon.lvclass out"=w203:refnum<class "Icon.lvclass">)  [unwired: 7 in]
      n79 = Bundle By Name(cluster=w204, "Class.Icon"=w203) -> (w201:T1)
      n80 = call <resource>:"DeselectLayer.vi"("error in (no error)"=w202, "Data in"=w201) -> ("error out"=w197:errorcluster, "Data out"=w198:T1)  [unwired: 8 out]
      n81 = call <resource>:"UpdateLayerView_ScrollbarChanged.vi"("error in"=w197, "Scrollbar Position"=0, "Data in"=w198) -> ("error out"=w195:errorcluster, "Data out"=w196:T1)  [unwired: 7 out]
    }
    frame "Merge Selected Layers" {
      n82 = Unbundle By Name(w256) -> ("Class.Icon"=w258:refnum<class "Icon.lvclass">, "Class.Layer"=w242:refnum<class "FakedArray.lvclass">)
      n83 = call-dynamic "GET_ActiveData.vi"("error in (no error)"=w239, "FakedArray in"=w242) -> ("error out"=w240:errorcluster, "Active Data []"=w238:i32[], "FakedArray out"=w241:refnum<class "FakedArray.lvclass">)  [unwired: 7 out]
      n84 = call-dynamic "GET_RowsCols.vi"("error in (no error)"=w240, "FakedArray.lvclass in"=w241) -> ("error out"=w250:errorcluster, "# Rows"=w249:i32)  [unwired: 8 out]
      n85 = call-dynamic "GET_UserLayers.vi"("error in (no error)"=w250, "Icon.lvclass in"=w258) -> ("error out"=w262:errorcluster, "All Layers"=w268:refnum<class "Layer.lvclass">[], "Icon.lvclass out"=w269:refnum<class "Icon.lvclass">)  [unwired: 7 out]
      n86 = call <resource>:"Reset layer template selection.vi"("error in (no error)"=w262, "Data in"=w256) -> ("error out"=w261:errorcluster, "Data out"=w255:T1)  [unwired: 1 in, 7 out]
      n87 = Sort 1D Array(array=w238) -> (sorted array=w275:i32[])
      n88 = call <resource>:"Separate Selected Layers.vi"("Active Indices"=w275, "All Layers"=w268) -> ("Layers out in Array"=w266:refnum<class "Layer.lvclass">[], "Layers out not in Array"=w267:refnum<class "Layer.lvclass">[])  [unwired: 8 out]
      n89 = Index Array(array=w275) -> (element=w247:i32)  [unwired: 1 in]
      n90 = call "Empty Picture"() -> ("empty picture"=w271:picture)
      n91 = for {
        shift-right: [w280] -> w273
        shift-left: w271 -> [w281]
        tunnel: w266 -> [w276] mode=indexing
        n92 = call-dynamic "GET_LayerData.vi"("Layer.lvclass in"=w276) -> ("Data"=w278:T11, "Origin"=w277:T5)  [unwired: 1 in, 8 out]
        n93 = Unbundle By Name(w278) -> ("Opacity"=w282:u8, "Visibility?"=w283:bool, "LayerIcon"=w279:picture)
        n94 = case shown="True" w283 {
          tunnel: w282 -> [_ w290]
          tunnel: w281 -> [w284 w289]
          tunnel: [w284 w288] -> w280
          tunnel: w279 -> [_ w287]
          tunnel: w277 -> [_ w286]
          frame False {
          }
          frame True {
            n95 = call <vilib>:"Draw Picture based on Origin.vi"("Origin"=w286, "LayerIcon in"=w287) -> ("LayerIcon out"=w285:picture)  [unwired: 1 in, 8 out]
            n96 = call <vilib>:"Apply Opacity.vi"("% (100)"=w290, "Bottom"=w289, "Top"=w285) -> ("new picture"=w288:picture)  [unwired: 8 out]
          }
        }
      }
      n97 = Bundle By Name(cluster=T11 {"LayerIcon"=bytes[0], "LayerName"="", "Opacity"=0, "Visibility?"=FALSE} ("Data"), "Opacity"=u8 100, "Visibility?"=TRUE, "LayerIcon"=w273, "LayerName"=w264) -> (w272:T11)
      n98 = call <vilib>:"Create default Layer.vi"() -> ("Layer.lvclass out"=w259:refnum<class "Layer.lvclass">)  [unwired: 1 in, 10 out]
      n99 = call-dynamic "SET_Layer_Data.vi"("error in (no error)"=w261, "Data"=w272, "Layer.lvclass in"=w259) -> ("error out"=w260:errorcluster, "Layer.lvclass out"=w270:refnum<class "Layer.lvclass">)  [unwired: 1 in, 6 out]
      n100 = Insert Into Array(array=w267, index=w247, new element=w270) -> (w265:refnum<class "Layer.lvclass">[])
      n101 = Subtract(x=w247, y=w249) -> (x-y=w248:i32)
      n102 = call-dynamic "SET_UserLayers.vi"("error in (no error)"=w260, "Layers"=w265, "Icon.lvclass in"=w269) -> ("error out"=w252:errorcluster, "Icon.lvclass out"=w257:refnum<class "Icon.lvclass">)  [unwired: 7 in]
      n103 = In Range and Coerce(upper limit=w247, x=w248, lower limit=0) -> (coerced(x)=w245:i32)  [unwired: 1 out]
      n104 = Bundle By Name(cluster=w255, "Class.Icon"=w257) -> (w254:T1)
      n105 = call <resource>:"UpdateLayerView_ScrollbarChanged.vi"("error in"=w252, "Scrollbar Position"=w245, "Data in"=w254) -> ("error out"=w251:errorcluster, "Data out"=w253:T1)  [unwired: 7 out]
    }
    frame "Import Glyph from File" {
      n106 = call <resource>:"Load Glyph from File.vi"("error in (no error)"=w296) -> ("error out"=w295:errorcluster, "file name"=w292:string, "Pic Out"=w293:picture, "Canceled?"=w294:bool)  [unwired: 7 in]
      n107 = case shown="False" w294 {
        tunnel: w299 -> [w304 w307]
        tunnel: [w305 w308] -> w298
        tunnel: [w303 w307] -> w297
        tunnel: w295 -> [w306 w308]
        tunnel: w293 -> [w301 _]
        tunnel: w292 -> [w302 _]
        tunnel: [TRUE _] -> w291
        frame False {
          n108 = call <resource>:"Create new layer_LayerName_Picture.vi"("error in"=w306, "Layer name"=w302, "Picture"=w301, "Data in"=w304) -> ("error out"=w305:errorcluster, "Data out"=w303:T1)  [unwired: 6 in]
        }
        frame True {
        }
      }
    }
    frame "Import Icon from Owning Library" {
      n109 = Unbundle By Name(w311) -> ("Class.Icon"=w319:refnum<class "Icon.lvclass">)
      n110 = call <resource>:"Read Data from Caller.vi"("error in (no error)"=w321) -> ("error out"=w318:errorcluster, "Library Icon"=w316:picture)  [unwired: 5 in, 4 out]
      n111 = call-dynamic "GET_UserLayers.vi"("error in (no error)"=w318, "Icon.lvclass in"=w319) -> ("error out"=w313:errorcluster, "All Layers"=w317:refnum<class "Layer.lvclass">[], "Icon.lvclass out"=w315:refnum<class "Icon.lvclass">)  [unwired: 7 out]
      n112 = call <resource>:"Create or Substitute NI_Layer layer.vi"("All Layers in"=w317, "new picture"=w316) -> ("All Layers out"=w314:refnum<class "Layer.lvclass">[])
      n113 = call-dynamic "SET_UserLayers.vi"("error in (no error)"=w313, "Layers"=w314, "Icon.lvclass in"=w315) -> ("error out"=w312:errorcluster, "Icon.lvclass out"=w310:refnum<class "Icon.lvclass">)  [unwired: 7 in]
      n114 = Bundle By Name(cluster=w311, "Class.Icon"=w310) -> (w309:T1)
    }
    frame "Redo", "Undo" {
      w345 = FALSE ("TM Set?")
      n115 = Unbundle By Name(w327) -> ("Class.Ants"=w326:refnum<class "Ants.lvclass">, "Ref.TextMarker"=w343:refnum<vi>)
      n116 = call <resource>:"Const Temp Coordinate 2 points.vi"() -> ("Const Temp Coordinate"=w346:T5)  [unwired: 11 out]
      n117 = call <resource>:"Const Temp Coordinate 4 points.vi"() -> ("Const Temp Coordinate"=w347:T21)  [unwired: 11 out]
      n118 = call "Empty Picture"() -> ("empty picture"=w344:picture)
      n119 = Bundle By Name(cluster=w327, "Support.Temp Icon"=w344, "Support.CTRL Pressed"=w345, "Support.Move Selection?"=w345, "Support.TM Set?"=w345, "Support.AntsRect"=w347, "Support.AntsRect Orig"=w347, "Support.Mouse Down Coords"=w346, "Support.Temp Coord"=w346) -> (w323:T1)
      n120 = Equal?(x=w340, y="Undo") -> (x = y?=w338:bool)
      n121 = property class="Str"(reference=w343, "Visible"=FALSE) -> ()  [unwired: 1 in, 2 out]
      n122 = Select(t=Undo_Redo_Action."Undo" ("Action"), s=w338, f=Undo_Redo_Action."Redo" ("Action")) -> (s? t:f=w335:T12)
      n123 = Unbundle By Name(w323) -> ("Ref.menu reference"=w322:refnum<k9>)
      n124 = call <resource>:"FireAntsEvent.vi"("error in (no error)"=w325, "Ants in"=w326) -> ("error out"=w341:errorcluster)  [unwired: 2 in, 7 out]
      n125 = call <resource>:"FGV_Undo Redo.vi"("Action"=w335, "error in"=w341, "menu reference"=w322) -> ("error out"=w334:errorcluster, "State Out"=w328:string)  [unwired: 2 in, 5 out]
      n126 = Unflatten From String(type=string[] [] ("appended array"), binary string=w328, error in (no error)=w334) -> (value=w332:string[], error out=w330:errorcluster)  [unwired: 2 in, 1 out]
      n127 = case shown="No Error" w330 {
        selector: w330 -> [w350 _]
        tunnel: w332 -> [w351 _]
        tunnel: [w352 _] -> w331
        tunnel: w323 -> [w349 w353]
        tunnel: [w348 w353] -> w324
        frame No Error {
          n128 = call <resource>:"Replay Data from History.vi"("error in (no error)"=w350, 10:"Data in"=w351, 11:"Data in"=w349) -> ("error out"=w352:errorcluster, "Data out"=w348:T1)  [unwired: 5 in, 2 out]
        }
        frame Error {
          # "Do not\npropagate\nerror."
        }
      }
    }
    frame "Select All" {
      w376 = T22 {"Left"=0, "Top"=0, "Right"=32, "Bottom"=32} ("Rectangle")
      n129 = Unbundle By Name(w369) -> ("Class.Icon"=w361:refnum<class "Icon.lvclass">, "Class.Ants"=w370:refnum<class "Ants.lvclass">, "Ref.Tools"=w366:refnum<vi>, "Ref.Ants"=w375:refnum<vi>)
      n130 = property class="Pict"(reference=w375, error in=w373, "Visible"=TRUE) -> (error out=w364:errorcluster)  [unwired: 1 out]
      n131 = property class="RadioBtnsControl (strict)"(reference=w366, error in=w364, "Value"=T13."Select" ("Value (Signaling)")) -> (error out=w365:errorcluster)  [unwired: 1 out]
      n132 = call <resource>:"Const Temp Coordinate 2 points.vi"() -> ("Const Temp Coordinate"=w372:T5)  [unwired: 11 out]
      n133 = call <resource>:"FireAntsEvent.vi"("error in (no error)"=w365, "Rectangle (default: deselect)"=w376, "Ants in"=w370) -> ("error out"=w362:errorcluster)  [unwired: 1 in, 7 out]
      n134 = Bundle By Name(cluster=w369, "Support.CTRL Pressed"=FALSE, "Support.Tool (old value)"=u32 111, "Support.Mouse Move Coords"=w372, "Support.Mouse Down Coords"=w372, "Support.AntsRect"=w376, "Support.AntsRect Orig"=w376) -> (w356:T1)
      n135 = call-dynamic "GET_All User Layers.vi"("error in (no error)"=w362, "Icon.lvclass in"=w361) -> ("error out"=w357:errorcluster, "User Layer"=w360:refnum<class "Layer.lvclass">[])  [unwired: 7 in, 1 out]
      n136 = Array Size(array=w360) -> (size(s)=w359:i32)
      n137 = for {
        N: w359 -> [_]
        tunnel: [w377] -> w358 mode=indexing
        i -> [w377]
      }
      n138 = call <resource>:"Set active Layer programmatically.vi"("error in"=w357, "Active Layer []"=w358, "Data in"=w356) -> ("error out"=w354:errorcluster, "Data out"=w355:T1)  [unwired: 7 in]
    }
    frame "Select Font", "Settings" {
      n139 = Equal?(x=w388, y="Select Font") -> (x = y?=w386:bool)
      n140 = Select(t="Text" ("y"), s=w386, f="") -> (s? t:f=w383:string)
      n141 = call <resource>:"IconEditorSettings.vi"("error in (no error)"=w378, "Active Tag"=w383, "Data in"=w381) -> ("error out"=w380:errorcluster, "Data out"=w379:T1)  [unwired: 7 out]
    }
    frame "Select None" {
      n142 = call <resource>:"Escape.vi"("error in"=w397, "Data in"=w396) -> ("error out"=w391:errorcluster, "Data out"=w392:T1)  [unwired: 2 in, 6 out]
      n143 = call <resource>:"DeselectLayer.vi"("error in (no error)"=w391, "Data in"=w392) -> ("error out"=w394:errorcluster, "Data out"=w393:T1)  [unwired: 8 out]
      n144 = call <resource>:"Reset layer template selection.vi"("error in (no error)"=w394, "Data in"=w393) -> ("error out"=w390:errorcluster, "Data out"=w389:T1)  [unwired: 1 in, 7 out]
    }
    frame "Show Terminals" {
      n145 = Unbundle By Name(w403) -> ("Class.Settings"=w404:refnum<class "Settings.lvclass">)
      n146 = call-dynamic "GET_Show.vi"("error in"=w399, "Settings.lvclass in"=w404) -> ("error out"=w410:errorcluster, "Show Terminals?"=w407:bool, "Settings.lvclass out"=w412:refnum<class "Settings.lvclass">)  [unwired: 7 out]
      n147 = Not(x=w407) -> (.not. x?=w408:bool)
      n148 = call <resource>:"ShowTerminals.vi"("Set Pic? (T)"=TRUE, "error in"=w410, "Tag enabled?"=TRUE, "Show Terminals?"=w408, "Data in"=w403) -> ("error out"=w409:errorcluster, "Data out"=w402:T1)  [unwired: 1 in, 4 out]
      n149 = call-dynamic "SET_Show.vi"("error in"=w409, "Show Terminals?"=w408, "Settings.lvclass in"=w412) -> ("error out"=w400:errorcluster, "Settings.lvclass out"=w401:refnum<class "Settings.lvclass">)  [unwired: 1 in, 6 out]
      n150 = Bundle By Name(cluster=w402, "Class.Settings"=w401) -> (w398:T1)
    }
    frame "Synchronize with Icon Library" {
      n151 = vi-ref <resource>:"ni.com_iconlibrary.vi"() -> (w424:refnum<vi>)
      n152 = property class="VI"(reference=w424, error in=w422) -> (error out=w421:errorcluster, "Path"=w423:path)  [unwired: 1 out]
      n153 = Open VI Reference(vi path=w423, error in (no error)=w421) -> (vi reference=w425:refnum<vi>, error out=w426:errorcluster)  [unwired: 4 in]
      n154 = invoke class="VI" method="Run VI"(reference=w425, error in=w426, "Wait until done"=TRUE ("Wait Until Done"), "Auto Dispose Ref"=FALSE ("Auto Dispose Reference")) -> (reference out=w417:refnum<vi>, error out=w418:errorcluster)  [unwired: 1 in, 3 out]
      n155 = Close Reference(reference=w417, error in (no error)=w418) -> (error out=w415:errorcluster)
      n156 = Unbundle By Name(w415) -> ("code"=w416:i32)
      n157 = case shown="0, Default" w416 {
        tunnel: [w435 errorcluster {"status"=FALSE, "code"=0, "source"=""} ("error out")] -> w429
        tunnel: w427 -> [w434 _]
        tunnel: w415 -> [w433 _]
        tunnel: w414 -> [w432 w437]
        tunnel: [w432 w437] -> w413
        frame 0, Default {
          n158 = Unbundle By Name(w432) -> ("Ref.GlyphLoadAnimation"=w430:refnum<vi>, "Ref.refreshGlyphs"=w431:refnum<vi>)
          n159 = call <resource>:"Launch Dynamically Load Graphics.vi"("User events"=w434, "Path"=Pathes."Glyphs", "error in (no error)"=w433, "button ref"=w431, "animatedDecoration ref"=w430) -> ("error out"=w435:errorcluster)  [unwired: 1 in, 5 out]
        }
        frame 1039 {
          # "VI was aborted"
        }
      }
    }
    frame "Template" {
      n160 = call <resource>:"DrawIcon.vi"("Tools"=Tools."Ellipse", "error in (no error)"=w445, "Data in"=w450) -> ("error out"=w457:errorcluster, "Icon"=w456:picture, "Data out"=w441:T1)  [unwired: 2 in, 4 out]
      n161 = call <resource>:"Read Data from Caller.vi"() -> ("Icon Editor Invoker Type"=w452:T23)  [unwired: 3 in, 8 out]
      n162 = call <resource>:"Specify Path Enum.vi"("Icon Editor Invoker Type"=w452) -> ("Path"=w451:T9)  [unwired: 10 out]
      n163 = call <vilib>:"Get LV Glyph Path.vi"("Path"=w451, "error in (no error)"=w457) -> ("error out"=w449:errorcluster, "Requested Path"=w446:path)  [unwired: 1 in, 7 out]
      n164 = call <vilib>:"Get Image Data.vi"("Pic In"=w456) -> ("image data out"=w455:T15)  [unwired: 3 in, 7 out]
      n165 = call <resource>:"Save Graphic.vi"("Loc string caption"=w442, "FP Title"=w447, "error in (no error)"=w449, "Start path in"=w446) -> ("error out"=w448:errorcluster, "Output"=w439:path)  [unwired: 6 out]
      n166 = Empty String/Path?(string/path=w439) -> (empty?=w443:bool)
      n167 = case shown="False" w443 {
        tunnel: w455 -> [w470 _]
        tunnel: w453 -> [w467 _]
        tunnel: w451 -> [w461 _]
        tunnel: w448 -> [w466 w474]
        tunnel: w439 -> [w460 _]
        tunnel: [w465 w474] -> w444
        tunnel: w441 -> [w464 w473]
        tunnel: [w464 w473] -> w440
        frame False {
          n168 = flat-sequence {
            tunnel: w460 -> [w472]
            tunnel: [w472] -> w459
            frame #0 {
              # "If the user pathologically deleted the specified folder while the dialog was up, this code will ensure that the owning folder exists when trying to save the .png file."
              n169 = Strip Path(path=w472) -> (stripped path=w471:path)  [unwired: 1 out]
              n170 = call <vilib>:"Create Directory Recursive.vi"("directory"=w471) -> ()  [unwired: 4 in, 3 out]
            }
          }
          n171 = Unbundle By Name(w464) -> ("Ref.TemplateLoadAnimation"=w463:refnum<vi>, "Ref.refreshTemplates"=w462:refnum<vi>)
          n172 = call <vilib>:"Write PNG File.vi"("error in (no error)"=w466, "image data"=w470, "path to PNG file"=w459) -> ("error out"=w469:errorcluster)  [unwired: 1 in, 7 out]
          n173 = call <resource>:"Launch Dynamically Load Graphics.vi"("User events"=w467, "Template saved?"=TRUE, "Path"=w461, "error in (no error)"=w469, "button ref"=w462, "animatedDecoration ref"=w463) -> ("error out"=w465:errorcluster)  [unwired: 5 out]
        }
        frame True {
        }
      }
    }
    frame Default {
    }
  }
  n174 = call <resource>:"ViewLayer.vi"("Add to Undo?"=w13, "error in (no error)"=w16, "Data in"=w14) -> ("error out"=w7:errorcluster, "Data out"=→"Data out":T1)  [unwired: 1 in, 6 out]
  n175 = call <resource>:"Defer_FP_Updates.vi"("Defer Panel Updates"=FALSE, "error in (no error)"=w7, "lv_icon.vi in"=w5) -> ("error out"=→"error out":errorcluster)  [unwired: 8 out]
